vi "Global-Stop (SubVI).vi"(1 "Mode (Read)":enum16{"Read", "Write"}(ring), 3 "IN":bool) -> (0 "OUT":bool)   [LabVIEW 2010]
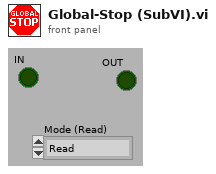
[diagram p1: front panel]
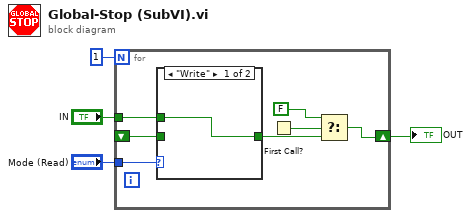
[diagram p0: block diagram]
diagram:
  n1 = for {
    N: 1 -> [_]
    shift-right: [w5] -> w1
    shift-left: _ -> [w10]
    tunnel: "Mode (Read)" -> [w11]
    tunnel: "IN" -> [w9]
    n2 = case shown="\"Write\"" w11 {
      tunnel: [w12 w13] -> w6
      tunnel: w10 -> [_ w13]
      tunnel: w9 -> [w12 _]
      frame "Write" {
      }
      frame "Read" {
      }
    }
    n3 = First Call?() -> (First Call?: T/F=w7:bool)
    n4 = Select(t=FALSE ("IN"), s=w7, f=w6) -> (s? t:f=w5:bool)
  }
  "OUT" <- w1
